vi "GoTo Tangent.vi"(4 "Passe":bool, 6 "Cone de chute":dbl=0.55 format="%#_13g", 7 "IA State Input in":T2, 8 "distance between ball and robot":dbl=250.0 format="%#_13g", 9 "Ball":dbl[](array[numeric])=[-1986.6092529296875, -3009.6396484375], 10 "Target":dbl[](array[numeric]), 11 "R":dbl[](array[numeric])=[-2840.578369140625, -1536.7857666015625, -1.0371381044387817]) -> (1 "Destination":dbl[](array[numeric]), 2 "Output\nVelocity":dbl[](array[numeric]) format="%.2f")   [LabVIEW 2017]
uses:
  Core/AI Input.ctl
  Core/AI Robot.ctl
  Intel/Functions Enum.ctl
  Intel/AttackerStates.ctl
  Path Planning/RRT/PathDests.ctl
  Path Planning/RRT/PathDest.ctl
  Core/AI Ball.ctl
  Core/Field Size.ctl
  Core/AI Judge.ctl
  Intel/Command Enum.ctl
  Util/Events/Events.ctl
  <vilib>/Analysis/coordinate.llb/Angle Range (Degree).ctl
  <vilib>/Analysis/coordinate.llb/Wrap Angle (scalar).vi
  <vilib>/Analysis/coordinate.llb/2D Cartesian Coordinate Rotation (Scalar).vi
  <vilib>/Analysis/NI_AALPro.lvlib
  <vilib>/Analysis/NI_AAL_Angle.lvlib
panel:
  in  "f":dbl[](array[numeric])=[0.0, 0.0, 0.0]
  in  "mag force\neps":dbl
  in  "angle range":T1=1 items=["none", "-180 to 180 (-pi to pi)", "0 to 360 (0 to 2pi)"]
  out "Waveform Chart 2":dbl[][](graph)
  out "Robot":dbl[](array[numeric])=[-2840.578369140625, -1536.7857666015625, -1.0371381044387817]
  out "Waveform Chart":dbl[][](graph)
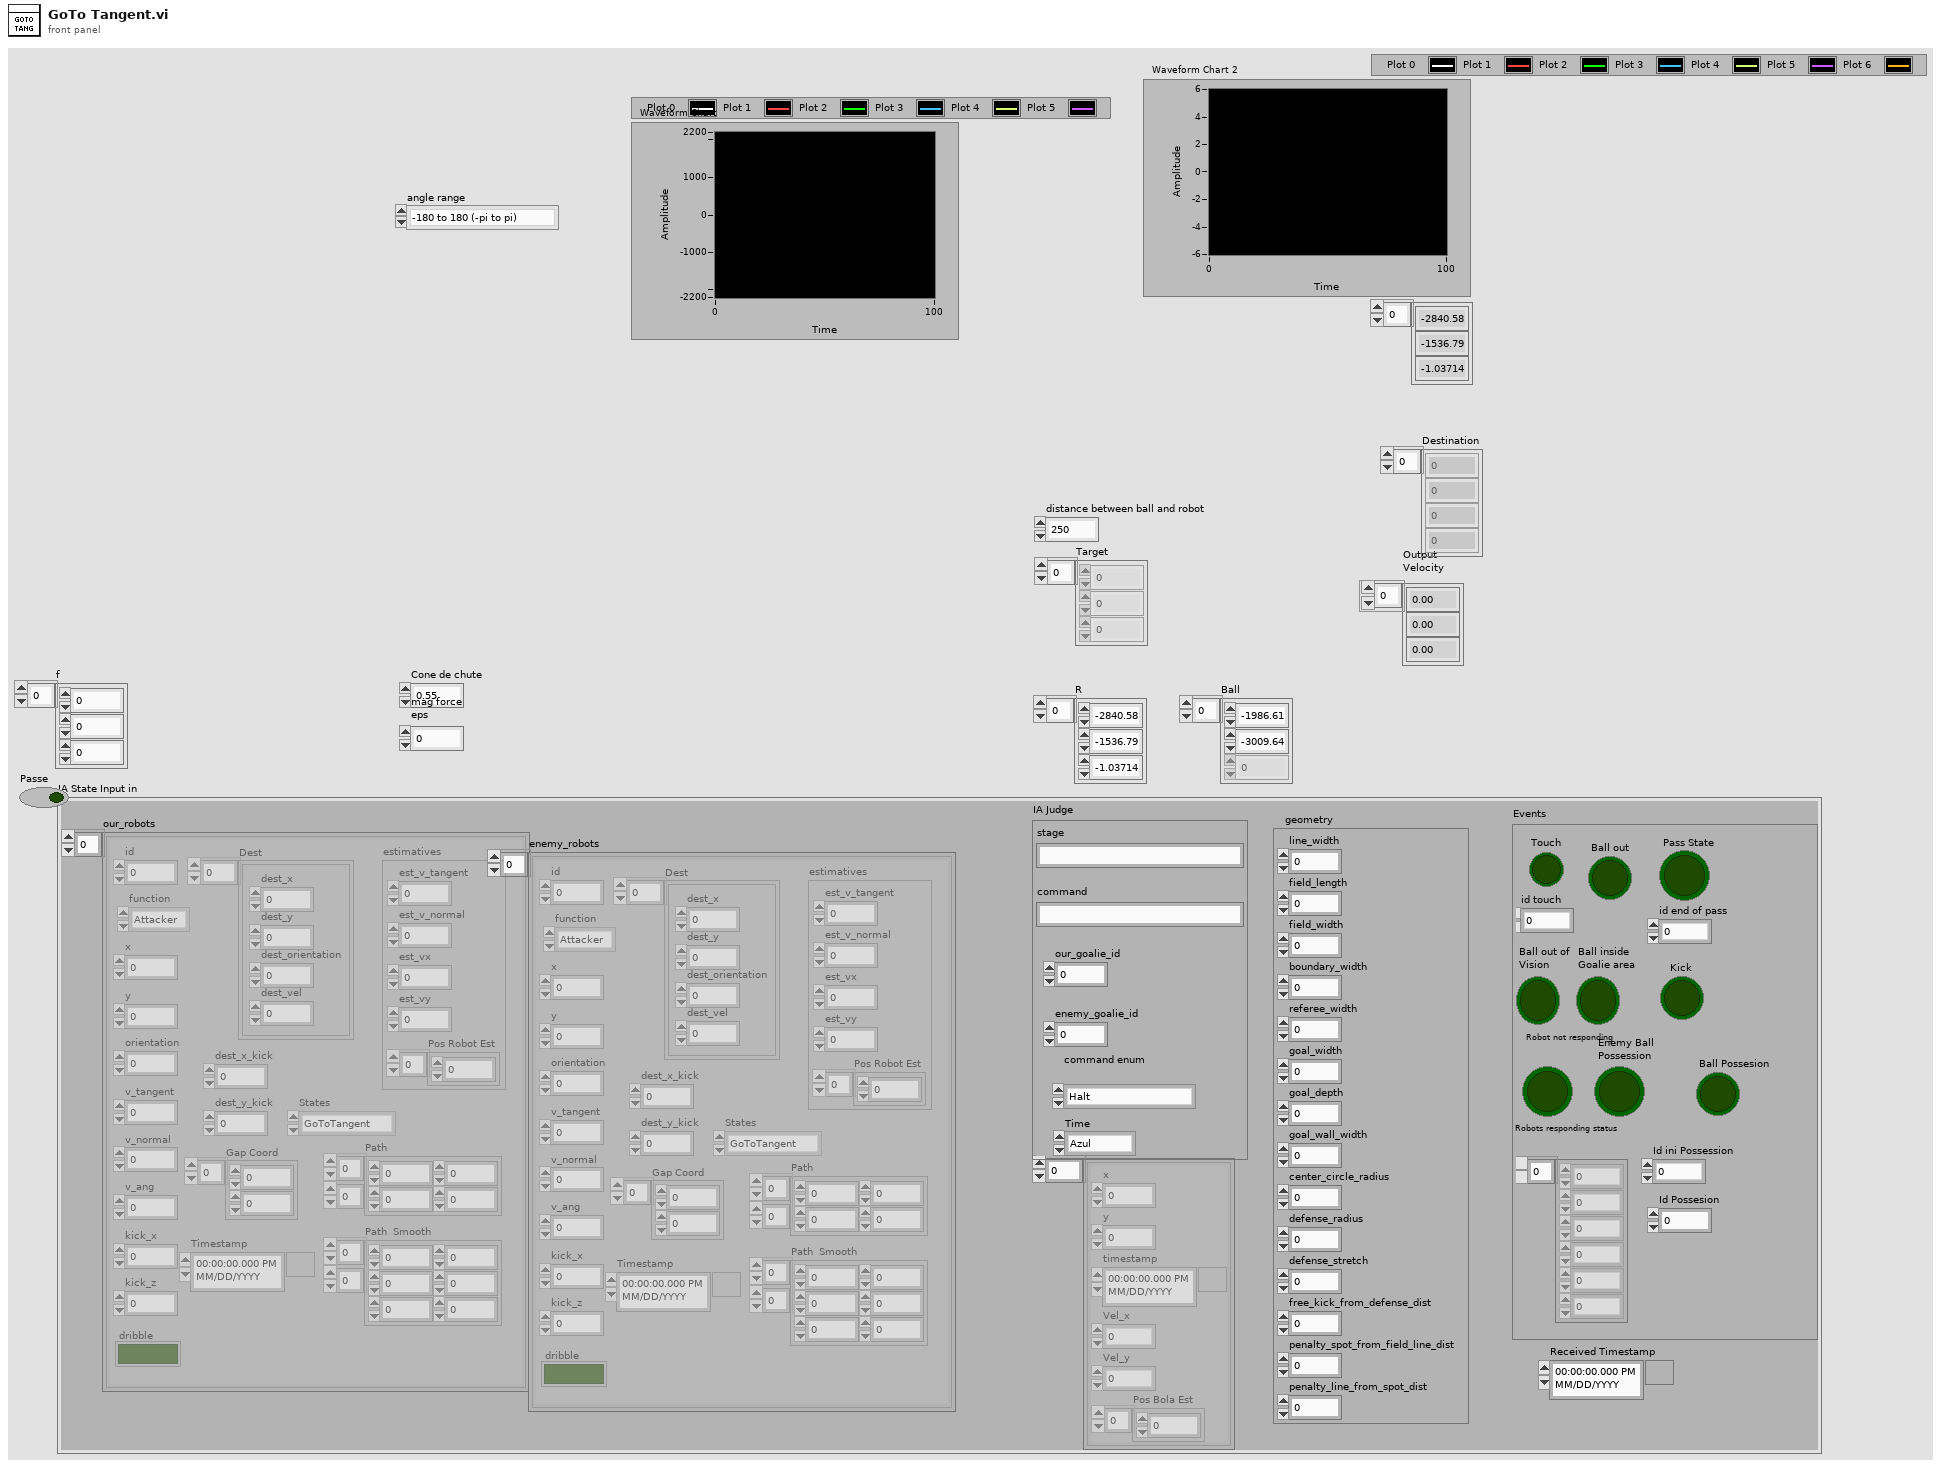
[diagram p1: front panel]
types:
  T1 = typedef "NI_AAL_Angle.lvlib/Angle Range (Degree).ctl" = u16
  T2 = typedef "AI Input.ctl" = cluster{"our_robots":T3[], "enemy_robots":T3[], "balls":T8[], "geometry":T9, "IA Judge":T10, "Received Timestamp":timestamp, "Events":T12}
  T3 = typedef "AI Robot.ctl" = cluster{"id":u32, "function":T4, "x":dbl, "y":dbl, "orientation":dbl, "v_tangent":dbl, "v_normal":dbl, "v_ang":dbl, "kick_x":dbl, "kick_z":dbl, "dribble":bool, "Timestamp":timestamp, "estimatives":cluster{"est_v_tangent":dbl, "est_v_normal":dbl, "est_vx":dbl, "est_vy":dbl, "Pos Robot Est":dbl[]}, "dest_x_kick":dbl, "dest_y_kick":dbl, "Gap Coord":dbl[], "States":T5, "Path ":dbl[][], "Path  Smooth":dbl[][], "Dest":T6}
  T4 = typedef "Functions Enum.ctl" = enum16{"Attacker", "Goalie", "Defender", "Striker", "Goto 0", "Dummy", "Kicker", "ZigZag"}
  T5 = typedef "AttackerStates.ctl" = enum16{"Pass", "GoToTangent", "BallGetting", "GoToKick", ""}
  T6 = typedef "PathDests.ctl" = T7[]
  T7 = typedef "PathDest.ctl" = cluster{"dest_x":dbl, "dest_y":dbl, "dest_orientation":dbl, "dest_vel":dbl}
  T8 = typedef "AI Ball.ctl" = cluster{"x":dbl, "y":dbl, "timestamp":timestamp, "Vel_x":dbl, "Vel_y":dbl, "Pos Bola Est":dbl[]}
  T9 = typedef "Field Size.ctl" = cluster{"line_width":u32, "field_length":u32, "field_width":u32, "boundary_width":u32, "referee_width":u32, "goal_width":u32, "goal_depth":u32, "goal_wall_width":u32, "center_circle_radius":u32, "defense_radius":u32, "defense_stretch":u32, "free_kick_from_defense_dist":u32, "penalty_spot_from_field_line_dist":u32, "penalty_line_from_spot_dist":u32}
  T10 = typedef "AI Judge.ctl" = cluster{"stage":string, "command":string, "our_goalie_id":dbl, "enemy_goalie_id":dbl, "command enum":T11, "Time":enum16{"Azul", "Amarelo"}}
  T11 = typedef "Command Enum.ctl" = enum16{"Halt", "Stop", "Force Start", "PKA Normal Start", "Prepare Kickoff Ally", "PKE Normal Start", "Prepare Kickoff Enemy", "Prepare Penalty Ally", "PPA Normal Start", "Prepare Penalty Enemy", "PPE Normal Start", "Direct Free Enemy", "Direct Free Ally", "Indirect Free Enemy", "Indirect Free Ally", "Timeout Enemy", "Timeout Ally", "Goal Enemy", "Goal Ally", "Ball Placement Enemy", "Ball Placement Ally", "Normal Half Time", "Extra Time Break", "Extra Half Time", "None", "Post Game"}
  T12 = typedef "Events.ctl" = cluster{"Touch":bool, "Ball out":bool, "id touch":dbl, "Ball out of \nVision":bool, "Ball inside \nGoalie area":bool, "Robot not responding":bool, "Robots responding status":dbl[], "Enemy Ball \nPossession":bool, "Pass State":bool, "id end of pass":dbl, "Kick":bool, "Id ini Possession":dbl, "Ball Possesion":bool, "Id Possesion":dbl}
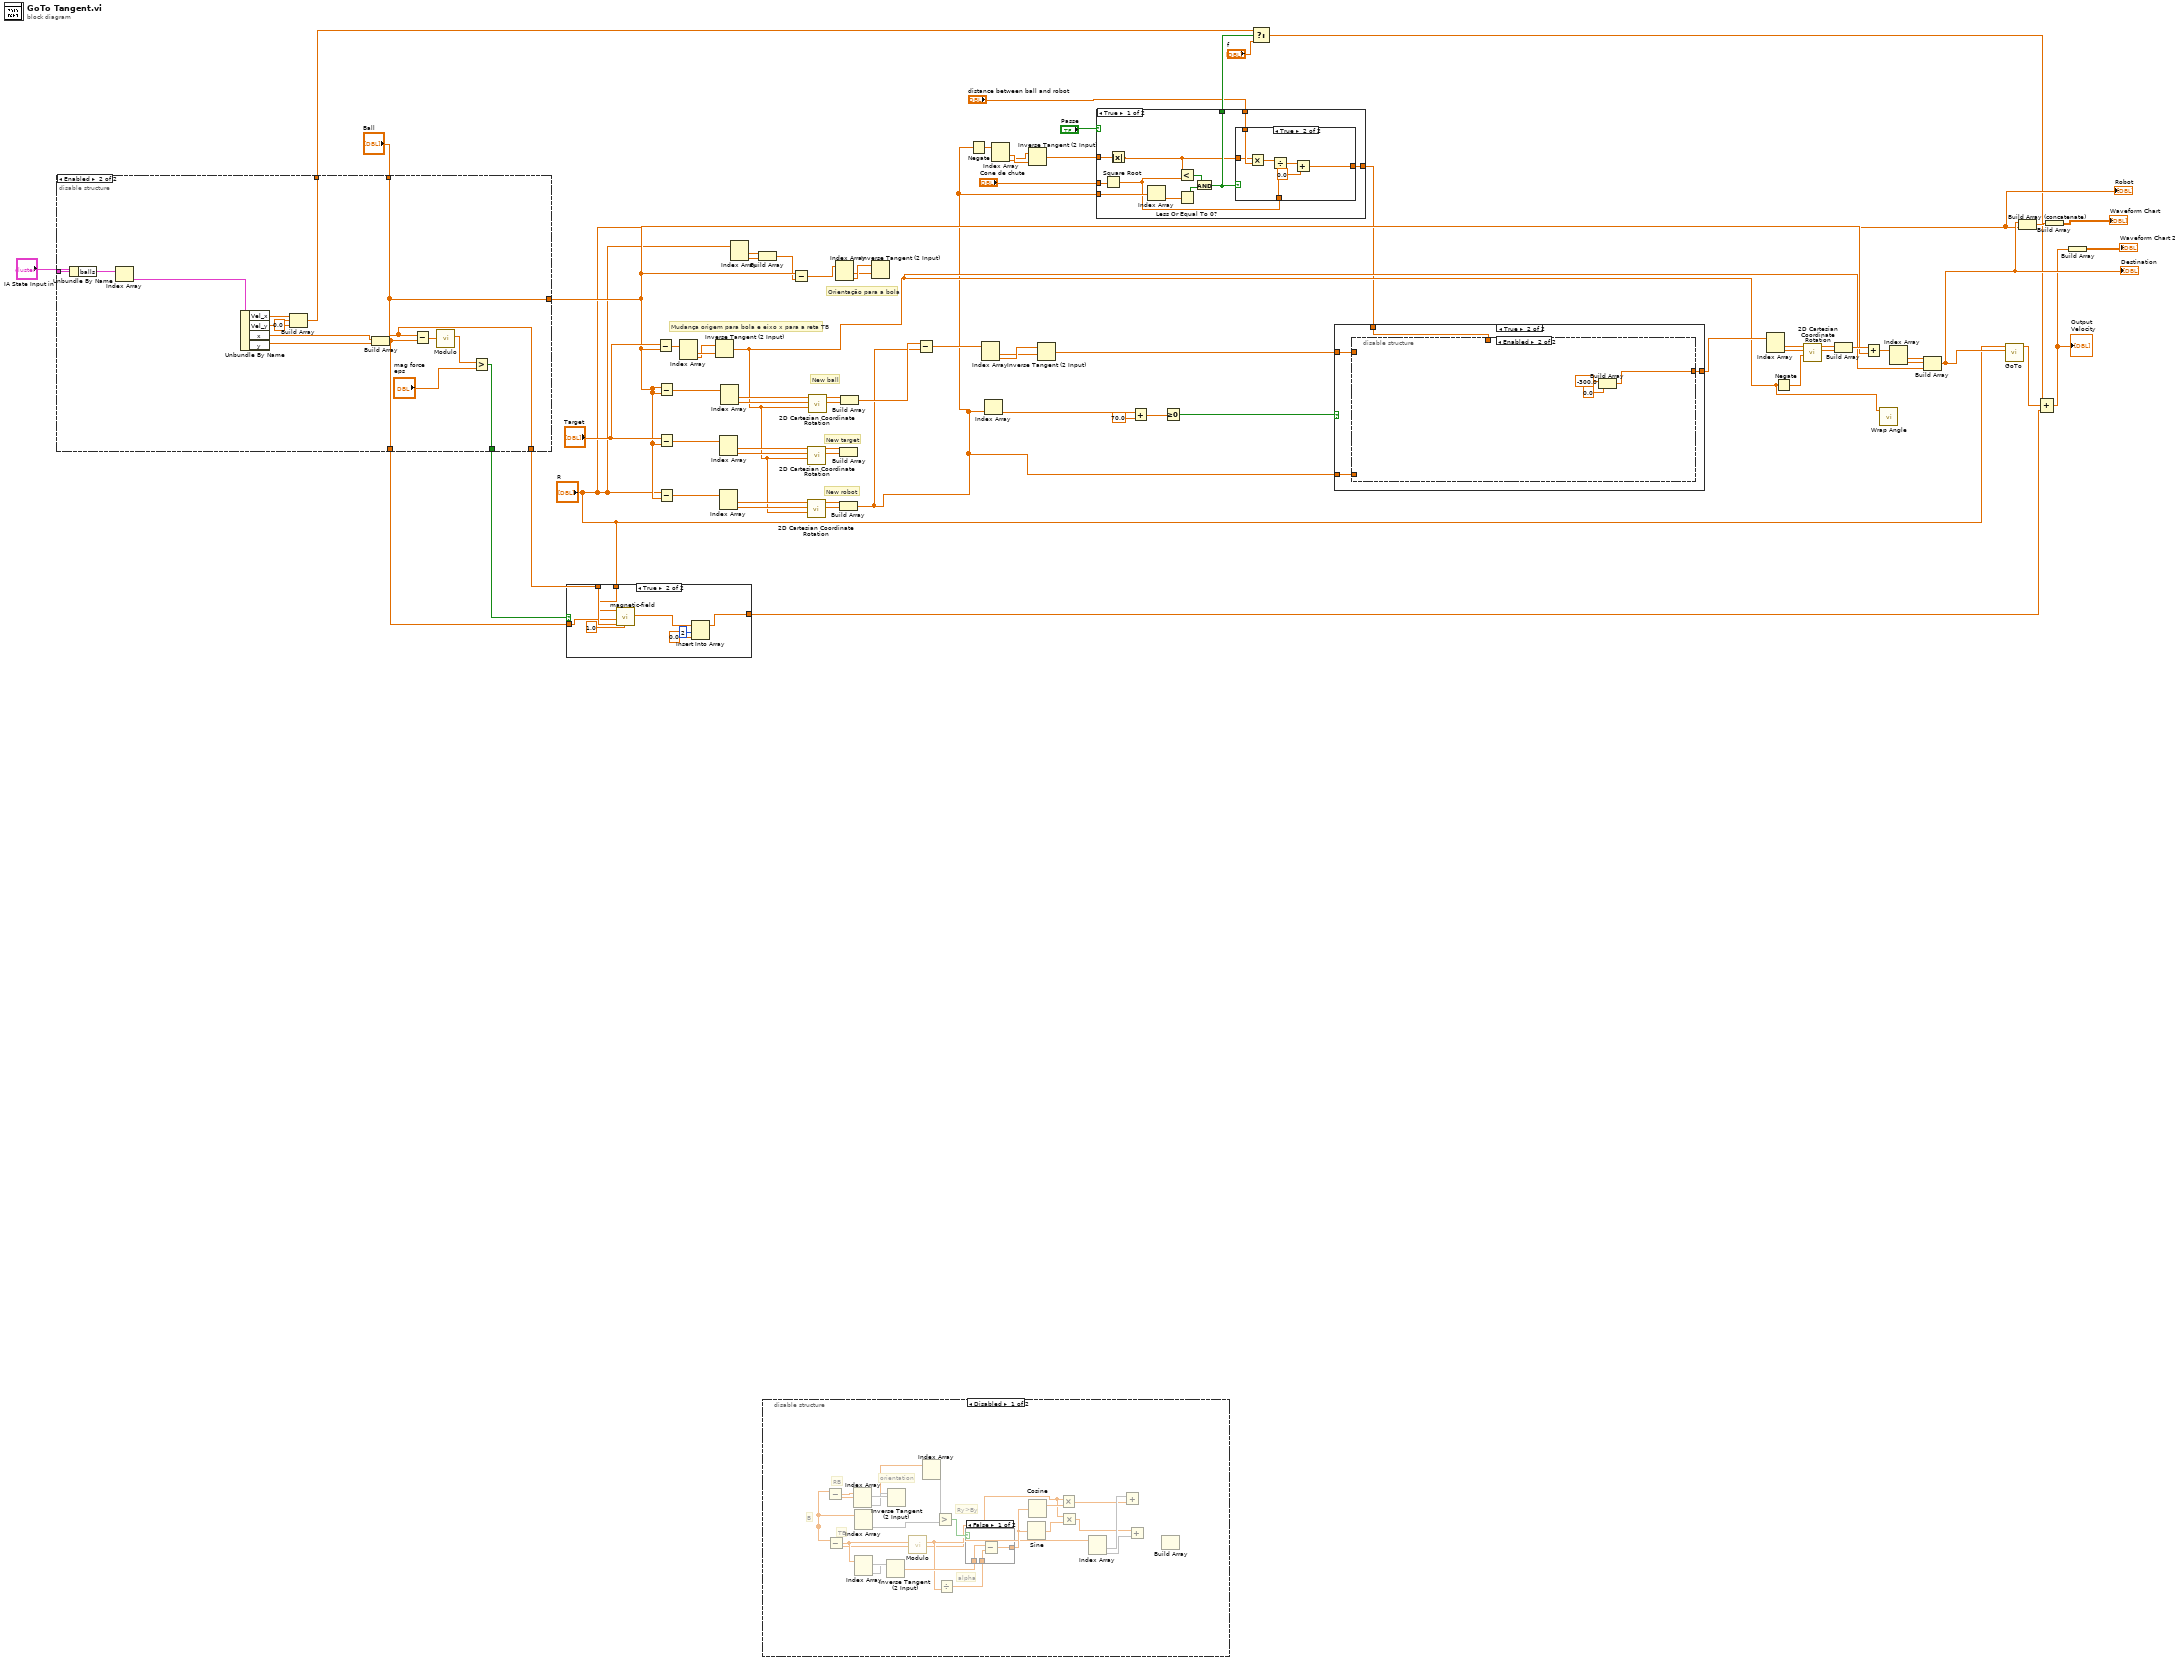
[diagram p0: block diagram]
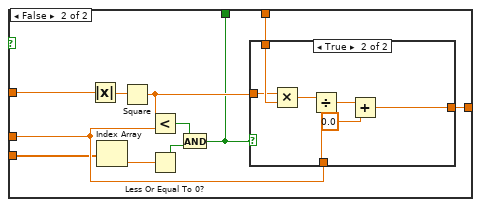
[diagram p3: hidden frame]
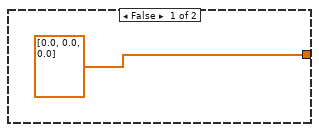
[diagram p5: hidden frame]
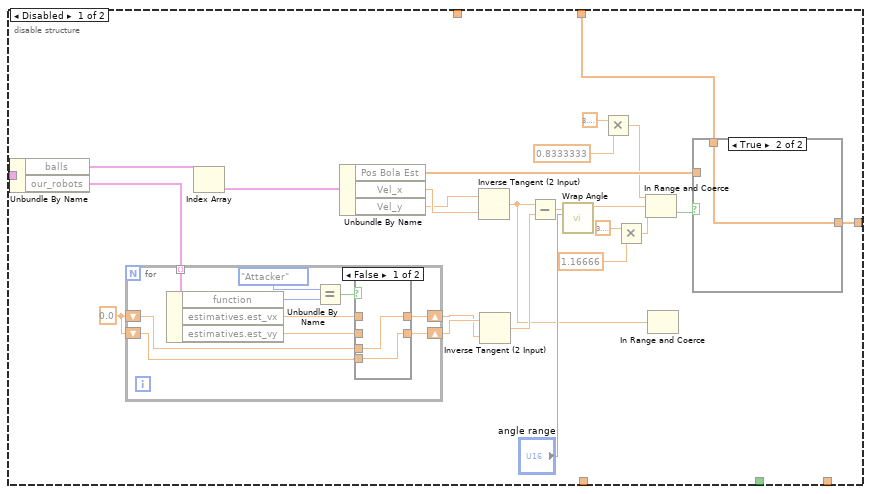
[diagram p6: hidden frame]
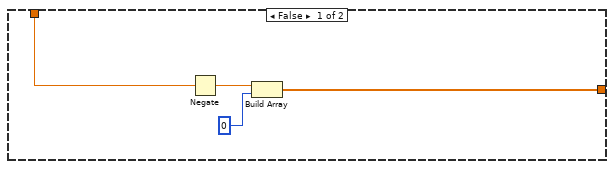
[diagram p9: hidden frame]
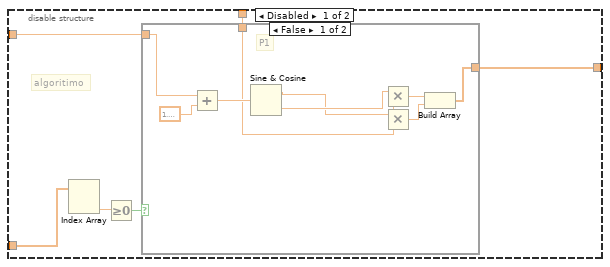
[diagram p10: hidden frame]
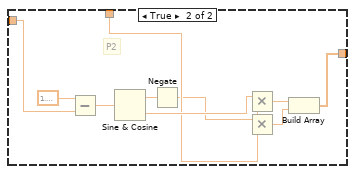
[diagram p11: hidden frame]
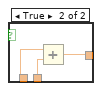
[diagram p12: hidden frame]
diagram:
  # "New ball"
  # "New target"
  # "New robot"
  # "Orientação para a bola"
  # "Mudança origem para bola e eixo x para a reta TB"
  n1 = disable-structure shown="Enabled" {
    disable-tunnel: [w96 w117] -> w31
    disable-tunnel: "IA State Input in" -> [w95 w126]
    disable-tunnel: "Ball" -> [w73 w117]
    disable-tunnel: [_ w118] -> w17
    disable-tunnel: [_ w117] -> w16
    disable-tunnel: [_ w116] -> w15
    disable-tunnel: [_ w114] -> w10
    frame Disabled {
      w91 = 0.0 ("est_vx")
      n2 = Unbundle By Name(w95) -> ("balls"=w94:T8[], "our_robots"=w92:T3[])
      n3 = for {
        tunnel: w92 -> [w106] mode=indexing
        shift-right: [w102] -> w88
        shift-left: w91 -> [w98]
        shift-right: [w99] -> w89
        shift-left: w91 -> [w97]
        n4 = Unbundle By Name(w106) -> ("function"=w104:T4, "estimatives.est_vx"=w101:dbl, "estimatives.est_vy"=w100:dbl)
        n5 = Equal?(x=Functions_Enum."Attacker" ("function"), y=w104) -> (x = y?=w105:bool)
        n6 = case shown="False" w105 {
          tunnel: [w108 w110] -> w102
          tunnel: w101 -> [_ w110]
          tunnel: w100 -> [_ w109]
          tunnel: [w107 w109] -> w99
          tunnel: w98 -> [w108 _]
          tunnel: w97 -> [w107 _]
          frame False {
          }
          frame True {
          }
        }
      }
      n7 = Index Array(array=w94) -> (element=w93:T8)  [unwired: 1 in]
      n8 = Unbundle By Name(w93) -> ("Pos Bola Est"=w90:dbl[], "Vel_x"=w87:dbl, "Vel_y"=w86:dbl)
      n9 = Inverse Tangent (2 Input)(1:w87, 2:w86) -> (0:w74:dbl)
      n10 = Inverse Tangent (2 Input)(1:w88, 2:w89) -> (0:w85:dbl)
      n11 = Subtract(x=w74, y=w85) -> (x-y=w83:dbl)
      n12 = call-poly <vilib>:"Wrap Angle.vi"("angle range"="angle range", "angle in"=w83) -> ("angle out"=w79:dbl)  [unwired: 8 in, 1 out]
      n13 = Multiply(x=3.141592653589793, y=0.8333333) -> (x*y=w76:dbl)
      n14 = Multiply(x=3.141592653589793, y=1.16666) -> (x*y=w82:dbl)
      n15 = In Range and Coerce(upper limit=w76, x=w79, lower limit=w82) -> (In Range?=w75:bool)  [unwired: 1 out]
      n16 = In Range and Coerce(x=w74) -> ()  [unwired: 2 in, 2 out]
      n17 = case shown="True" w75 {
        tunnel: [_ w111] -> w96
        tunnel: w90 -> [_ _]
        tunnel: w73 -> [_ w111]
        frame False {
        }
        frame True {
        }
      }
    }
    frame Enabled {
      n18 = Unbundle By Name(w126) -> ("balls"=w124:T8[])
      n19 = Index Array(array=w124) -> (element=w125:T8)  [unwired: 1 in]
      n20 = Unbundle By Name(w125) -> ("Vel_x"=w115:dbl, "Vel_y"=w113:dbl, "x"=w123:dbl, "y"=w122:dbl)
      n21 = Build Array(w115, w113, 0.0 ("element")) -> (w114:dbl[])
      n22 = Build Array(w123, w122) -> (w116:dbl[])
      n23 = Subtract(x=w117, y=w116) -> (x-y=w121:dbl[])
      n24 = call "Modulo.vi"("2D vector"=w121) -> ("Modulo"=w120:dbl)  [unwired: 10 in]
      n25 = Greater?(x=w120, y="mag force\neps") -> (0:w118:bool)
    }
  }
  n26 = case shown="True" w17 {
    tunnel: w16 -> [_ w134]
    tunnel: w15 -> [_ w133]
    tunnel: "R" -> [_ w132]
    tunnel: [dbl[] [0.0, 0.0, 0.0] ("magnetic force") w129] -> w13
    frame False {
    }
    frame True {
      n27 = call "magnetic-field.vi"("max force"=1.0, "goal pos"=w134, "enemy pos"=w133, "ally pos"=w132) -> ("magnetic force"=w130:dbl[])  [unwired: 7 in]
      n28 = Insert Into Array(array=w130, index=2, new element=0.0 ("new element/subarray")) -> (w129:dbl[])
    }
  }
  n29 = Subtract(x="Target", y=w31) -> (x-y=w63:dbl[])
  n30 = Subtract(x=w31, y=w31) -> (x-y=w70:dbl[])
  n31 = Subtract(x="Target", y=w31) -> (x-y=w67:dbl[])
  n32 = Subtract(x="R", y=w31) -> (x-y=w64:dbl[])
  n33 = Index Array(array=w63) -> (element #1=w62:dbl, element #2=w61:dbl)  [unwired: 2 in]
  n34 = Inverse Tangent (2 Input)(1:w62, 2:w61) -> (0:w25:dbl)
  n35 = Index Array(array=w64) -> (element #1=w66:dbl, element #2=w65:dbl)  [unwired: 2 in]
  n36 = Index Array(array=w67) -> (element #1=w69:dbl, element #2=w68:dbl)  [unwired: 2 in]
  n37 = Index Array(array=w70) -> (element #1=w72:dbl, element #2=w71:dbl)  [unwired: 2 in]
  n38 = Index Array(array="R") -> (element #1=w30:dbl, element #2=w29:dbl)  [unwired: 2 in]
  n39 = Build Array(w30, w29) -> (w28:dbl[])
  n40 = disable-structure shown="Disabled" {
    frame Disabled {
      # "Ry>By"
      # "orientation"
      # "RB"
      # "alpha"
      # "TB"
      # "B"
      n41 = Index Array() -> (array=w141:dbl[], element #2=w147)  [unwired: 2 in, 1 out]
      n42 = Index Array() -> (array=w137:dbl[], element #2=w148)  [unwired: 2 in, 1 out]
      n43 = Subtract(x=w141, y=w137) -> (x-y=w155:dbl)
      n44 = Index Array(array=w155) -> (element #1=w157, element #2=w156)  [unwired: 2 in]
      n45 = Inverse Tangent (2 Input)(1:w157, 2:w156) -> (0:w154:dbl)
      n46 = Greater?(x=w148, y=w147) -> (0:w146:bool)
      n47 = Index Array() -> (array=w136:dbl[], element #1=w144, element #2=w139)  [unwired: 2 in]
      n48 = Subtract(x=w141, y=w136) -> (x-y=w159:dbl)
      n49 = Index Array(array=w159) -> (element #1=w161, element #2=w160)  [unwired: 2 in]
      n50 = Inverse Tangent (2 Input)(1:w161, 2:w160) -> (0:w153:dbl)
      n51 = call "Modulo.vi"("2D vector"=w159) -> ("Modulo"=w145:dbl)  [unwired: 10 in]
      n52 = Divide(y=w145) -> (x=w158:dbl, x/y=w152:dbl)
      n53 = case shown="False" w146 {
        tunnel: w153 -> [w163 w167]
        tunnel: w152 -> [w164 w166]
        tunnel: [w162 w165] -> w151
        frame False {
          n54 = Subtract(x=w163, y=w164) -> (x-y=w162:dbl)
        }
        frame True {
          n55 = Add(x=w167, y=w166) -> (x+y=w165:dbl)
        }
      }
      n56 = Sine(x=w151) -> (sin(x)=w149:dbl)
      n57 = Cosine(x=w151) -> (cos(x)=w150:dbl)
      n58 = Multiply(x=w145, y=w150) -> (x*y=w143:dbl)
      n59 = Multiply(x=w145, y=w149) -> (x*y=w140:dbl)
      n60 = Add(x=w144, y=w143) -> (x+y=w142:dbl)
      n61 = Add(x=w140, y=w139) -> (x+y=w138:dbl)
      n62 = Build Array() -> ()  [unwired: 3 in, 1 out]
    }
    frame Enabled {
    }
  }
  n63 = Subtract(x=w31, y=w28) -> (x-y=w43:dbl[])
  n64 = call-poly <vilib>:"2D Cartesian Coordinate Rotation.vi"("theta"=w25, "y"=w65, "x"=w66) -> ("y out"=w55:dbl, "x out"=w56:dbl)  [unwired: 6 in, 1 out]
  n65 = call-poly <vilib>:"2D Cartesian Coordinate Rotation.vi"("theta"=w25, "y"=w68, "x"=w69) -> ("y out"=w59:dbl, "x out"=w60:dbl)  [unwired: 6 in, 1 out]
  n66 = call-poly <vilib>:"2D Cartesian Coordinate Rotation.vi"("theta"=w25, "y"=w71, "x"=w72) -> ("y out"=w57:dbl, "x out"=w58:dbl)  [unwired: 6 in, 1 out]
  n67 = Index Array(array=w43) -> (element #1=w44:dbl, element #2=w45:dbl)  [unwired: 2 in]
  n68 = Build Array(w56, w55) -> (w18:dbl[])
  n69 = Build Array(w60, w59) -> ()  [unwired: 1 out]
  n70 = Build Array(w58, w57) -> (w38:dbl[])
  n71 = Inverse Tangent (2 Input)(1:w44, 2:w45) -> ()  [unwired: 1 out]
  n72 = Subtract(x=w38, y=w18) -> (x-y=w52:dbl[])
  n73 = Negate(x=w18) -> (-x=w24:dbl[])
  n74 = Index Array(array=w52) -> (element #1=w53:dbl, element #2=w54:dbl)  [unwired: 2 in]
  n75 = Index Array(array=w18) -> (element=w2:dbl)  [unwired: 1 in]
  n76 = Index Array(array=w24) -> (element #1=w23:dbl, element #2=w22:dbl)  [unwired: 2 in]
  n77 = Inverse Tangent (2 Input)(1:w23, 2:w22) -> (0:w21:dbl)
  n78 = Inverse Tangent (2 Input)(1:w53, 2:w54) -> (0:w39:dbl)
  n79 = case shown="True" "Passe" {
    tunnel: w21 -> [w178 w197]
    tunnel: "Cone de chute" -> [w170 w196]
    tunnel: [w177 w195] -> w19
    tunnel: "distance between ball and robot" -> [w176 w194]
    tunnel: w18 -> [w175 w191]
    tunnel: [w171 w187] -> w9
    frame True {
      n80 = Square Root(x=w170) -> (sqrt(x)=w168:dbl)
      n81 = Absolute Value(x=w178) -> (abs(x)=w169:dbl)
      n82 = Index Array(array=w175) -> (element=w174:dbl)  [unwired: 1 in]
      n83 = Less?(x=w169, y=w168) -> (x < y?=w173:bool)
      n84 = Less Or Equal To 0?(x=w174) -> (x <= 0?=w172:bool)
      n85 = And(x=w173, y=w172) -> (x .and. y?=w171:bool)
      n86 = case shown="True" w171 {
        tunnel: w168 -> [_ w184]
        tunnel: [w179 w183] -> w177
        tunnel: w176 -> [w179 w182]
        tunnel: w169 -> [_ w181]
        frame False {
        }
        frame True {
          n87 = Multiply(x=w181, y=w182) -> (x*y=w186:dbl)
          n88 = Divide(x=w186, y=w184) -> (x/y=w185:dbl)
          n89 = Add(x=w185, y=0.0) -> (x+y=w183:dbl)
        }
      }
    }
    frame False {
      n90 = Absolute Value(x=w197) -> (abs(x)=w193:dbl)
      n91 = Index Array(array=w191) -> (element=w190:dbl)  [unwired: 1 in]
      n92 = Square(x=w193) -> (x^2=w192:dbl)
      n93 = Less?(x=w192, y=w196) -> (x < y?=w189:bool)
      n94 = Less Or Equal To 0?(x=w190) -> (x <= 0?=w188:bool)
      n95 = And(x=w189, y=w188) -> (x .and. y?=w187:bool)
      n96 = case shown="True" w187 {
        tunnel: w196 -> [_ w203]
        tunnel: [w198 w202] -> w195
        tunnel: w194 -> [w198 w201]
        tunnel: w192 -> [_ w200]
        frame False {
        }
        frame True {
          n97 = Multiply(x=w200, y=w201) -> (x*y=w205:dbl)
          n98 = Divide(x=w205, y=w203) -> (x/y=w204:dbl)
          n99 = Add(x=w204, y=0.0) -> (x+y=w202:dbl)
        }
      }
    }
  }
  n100 = Add(x=w2, y=70.0) -> (x+y=w1:dbl)
  n101 = Greater Or Equal To 0?(x=w1) -> (x >= 0?=w4:bool)
  n102 = Select(t=w10, s=w9, f="f") -> (s? t:f=w7:dbl[])
  n103 = case shown="True" w4 {
    tunnel: w39 -> [_ w213]
    tunnel: [w208 w212] -> w47
    tunnel: w18 -> [_ w211]
    tunnel: w19 -> [w206 w210]
    frame False {
      n104 = Negate(x=w206) -> (-x=w207:dbl)
      n105 = Build Array(w207, 0 ("index")) -> (w208:dbl[])
    }
    frame True {
      n106 = disable-structure shown="Enabled" {
        disable-tunnel: w213 -> [w218 _]
        disable-tunnel: [w217 w241] -> w212
        disable-tunnel: w211 -> [w215 _]
        disable-tunnel: w210 -> [w214 _]
        frame Disabled {
          # "algoritimo"
          n107 = Index Array(array=w215) -> (element #2=w219:dbl)  [unwired: 2 in, 1 out]
          n108 = Greater Or Equal To 0?(x=w219) -> (x >= 0?=w216:bool)
          n109 = case shown="False" w216 {
            tunnel: w218 -> [w223 w232]
            tunnel: [w225 w235] -> w217
            tunnel: w214 -> [w221 w231]
            frame False {
              # "P1"
              n110 = Add(x=w223, y=1.5707963267948966) -> (x+y=w224:dbl)
              n111 = Sine & Cosine(0:w224) -> (1:w220:dbl, 2:w226:dbl)
              n112 = Multiply(x=w226, y=w221) -> (x*y=w228:dbl)
              n113 = Multiply(x=w220, y=w221) -> (x*y=w227:dbl)
              n114 = Build Array(w228, w227) -> (w225:dbl[])
            }
            frame True {
              # "P2"
              n115 = Subtract(x=1.5707963267948966, y=w232) -> (x-y=w234:dbl)
              n116 = Sine & Cosine(0:w234) -> (1:w230:dbl, 2:w238:dbl)
              n117 = Negate(x=w230) -> (-x=w229:dbl)
              n118 = Multiply(x=w238, y=w231) -> (x*y=w236:dbl)
              n119 = Multiply(x=w229, y=w231) -> (x*y=w237:dbl)
              n120 = Build Array(w236, w237) -> (w235:dbl[])
            }
          }
        }
        frame Enabled {
          n121 = Build Array(-300.0 ("element"), 0.0 ("element")) -> (w241:dbl[])
        }
      }
    }
  }
  n122 = Index Array(array=w47) -> (element #1=w51:dbl, element #2=w50:dbl)  [unwired: 2 in]
  n123 = Negate(x=w25) -> (-x=w36:dbl)
  n124 = call-poly <vilib>:"2D Cartesian Coordinate Rotation.vi"("theta"=w36, "y"=w50, "x"=w51) -> ("y out"=w48:dbl, "x out"=w49:dbl)  [unwired: 6 in, 1 out]
  n125 = Build Array(w49, w48) -> (w46:dbl[])
  n126 = Add(x=w46, y=w31) -> (x+y=w42:dbl[])
  n127 = call-poly <vilib>:"Wrap Angle.vi"("angle in"=w25) -> ()  [unwired: 9 in, 2 out]
  n128 = Index Array(array=w42) -> (element #1=w41:dbl, element #2=w40:dbl)  [unwired: 2 in]
  n129 = Build Array(w41, w40, w25) -> (w37:dbl[])
  "Destination" <- w37
  n130 = call "GoTo.vi"("Target"=w37, "Position"="R") -> ("Output\nVelocity"=w12:dbl[])  [unwired: 8 in, 1 out]
  n131 = Build Array (concatenate)(w37, "R") -> (w35:dbl[])
  n132 = Compound Arithmetic op=ADD(w7, w12, w13) -> (w11:dbl[])
  "Output\nVelocity" <- w11
  n133 = Build Array(w35) -> (→"Waveform Chart":dbl[][])
  n134 = Build Array(w11) -> (→"Waveform Chart 2":dbl[][])
  "Robot" <- "R"
